vi "FIR_downsample_10.vi"(7 "reset":bool, 8 "valid in":bool, 10 "Q in":fxp<+/-,25,19>, 11 "I in":fxp<+/-,25,19>) -> (0 "valid out":bool, 2 "Q out":fxp<+/-,16,16>, 3 "I out":fxp<+/-,16,16>, 4 "ready for input":bool)   [LabVIEW 2013]
uses:
  <vilib>/rvi/FXPMathLib/FxpConvert/subVIs/nifxpmath_Convert_SimConfig.ctl
  <vilib>/fxp/LVFixedPointQuantizationPolicyTypeDef.ctl
  <vilib>/fxp/LVFixedPointOverflowPolicyTypeDef.ctl
  <vilib>/rvi/IPIntegrationNode/IPINode_Utilities/niFpgaIPINodeSimCore.vi
  <vilib>/rvi/FXPMathLib/FxpConvert/simVIs/DllFxpConvertTemp_sub.vi
  <vilib>/rvi/FXPMathLib/FxpInterpret/XNode/nifxpmath_Interpret.xnode
  <vilib>/rvi/XilinxIP/XIPIN_XNode/niFpgaXIPIN.xnode
  FIR_downsample_10/FIR downsample 10/FIR_downsample_10_3EB4078EBDC7483EBD6633791A17D2B3.dll
  <vilib>/rvi/IPIntegrationNode/IPINode_Xnode/niFpgaIPINode.xnode
  <vilib>/rvi/FXPMathLib/FxpConvert/XNode/nifxpmath_Convert.xnode
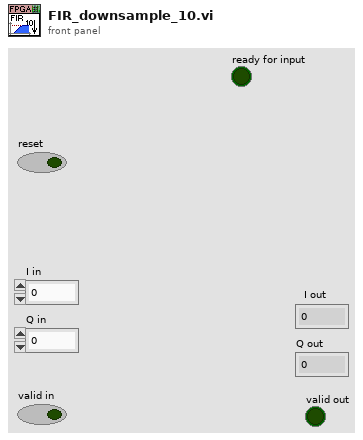
[diagram p1: front panel]
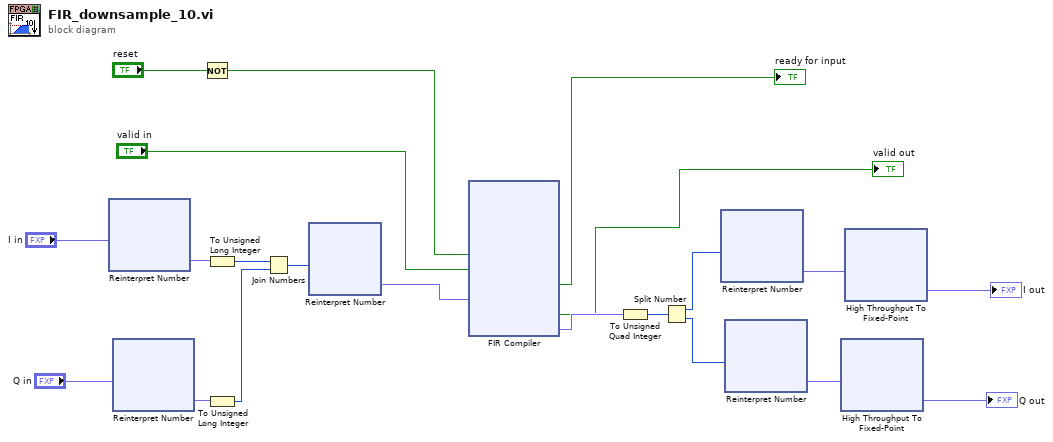
[diagram p0: block diagram]
diagram:
  n1 = xnode "Reinterpret Number"("x"="I in") -> ("y"=w9:fxp<+,25,25>)
  n2 = xnode "Reinterpret Number"("x"="Q in") -> ("y"=w7:fxp<+,25,25>)
  n3 = Not(x="reset") -> (.not. x?=w1:bool)
  n4 = To Unsigned Long Integer(number=w9) -> (unsigned 32bit integer=w8:u32)
  n5 = To Unsigned Long Integer(number=w7) -> (unsigned 32bit integer=w6:u32)
  n6 = Join Numbers(hi=w8, lo=w6) -> ((hi.lo)=w21:u64)
  n7 = xnode "Reinterpret Number"("x"=w21) -> ("y"=w18:fxp<+,64,64>)
  n8 = xnode ("FIR Compiler")("aresetn"=w1, "s_axis_data_tvalid"="valid in", "s_axis_data_tdata"=w18) -> ("s_axis_data_tready"=→"ready for input":bool, "m_axis_data_tvalid"=→"valid out":bool, "m_axis_data_tdata"=w5:fxp<+,64,64>)  [unwired: 1 in]
  n9 = To Unsigned Quad Integer(1:w5) -> (0:w14:u64)
  n10 = Split Number(x=w14) -> (hi(x)=w15:u32, lo(x)=w16:u32)
  n11 = xnode "Reinterpret Number"("x"=w15) -> ("y"=w12:fxp<+/-,32,20>)
  n12 = xnode "Reinterpret Number"("x"=w16) -> ("y"=w13:fxp<+/-,32,20>)
  n13 = xnode "High Throughput To Fixed-Point"("x"=w13) -> ("y"=→"Q out":fxp<+/-,16,16>)
  n14 = xnode "High Throughput To Fixed-Point"("x"=w12) -> ("y"=→"I out":fxp<+/-,16,16>)
